vi "add new data to graph.vi"(4 "New Timestamps":timestamp[](array[timestamp]), 7 "Data Array":dbl[](array[numeric]), 8 "Clear Graph":bool, 9 "Max Number of Datapoints":dbl=10000.0 format="%#_13g", 10 "Graph Data":T1(array[cluster])) -> (3 "Graph Data 2":T1(array[cluster]))   [LabVIEW 2013]
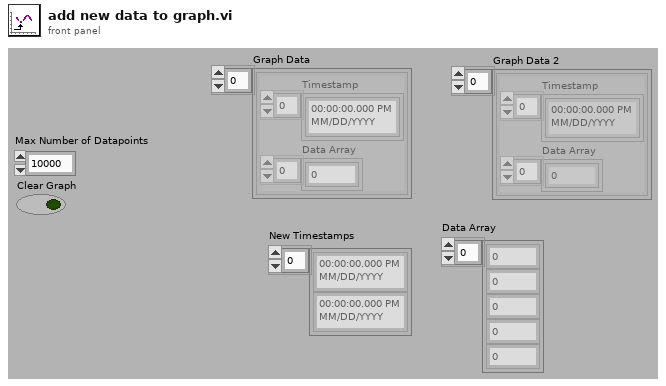
[diagram p1: front panel]
types:
  T1 = cluster{"Timestamp":timestamp[], "Data Array":dbl[]}[]
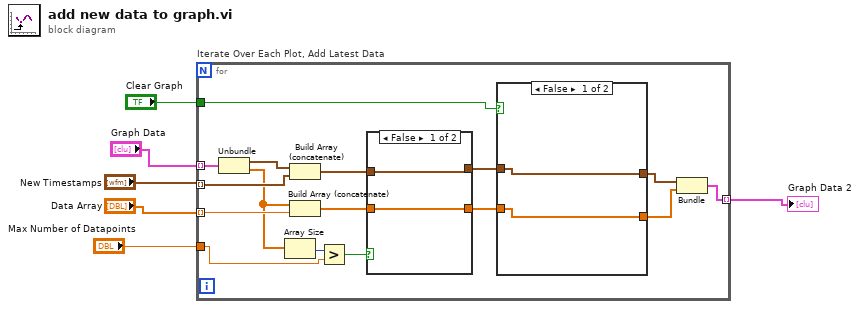
[diagram p0: block diagram]
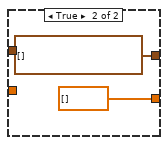
[diagram p2: hidden frame]
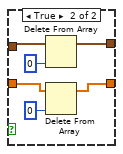
[diagram p3: hidden frame]
diagram:
  n1 = for "Iterate Over Each Plot, Add Latest Data" {
    tunnel: "Graph Data" -> [w22] mode=indexing
    tunnel: "New Timestamps" -> [w18] mode=indexing
    tunnel: "Data Array" -> [w20] mode=indexing
    tunnel: "Max Number of Datapoints" -> [w16]
    tunnel: "Clear Graph" -> [w14]
    tunnel: [w8] -> w5 mode=indexing
    n2 = Unbundle ("Split x and y")(w22) -> ("Timestamp"=w21:timestamp[], "Data Array"=w11:dbl[])
    n3 = Array Size(array=w11) -> (size(s)=w17:i32)
    n4 = Build Array (concatenate) ("Append Latest Values")(w21, w18) -> (w7:timestamp[])
    n5 = Build Array (concatenate)(w11, w20) -> (w19:dbl[])
    n6 = Greater?(x=w17, y=w16) -> (0:w15:bool)
    n7 = case shown="False" w15 {
      tunnel: w19 -> [w27 w32]
      tunnel: w7 -> [w28 w34]
      tunnel: [w28 w30] -> w13
      tunnel: [w27 w29] -> w12
      frame False {
      }
      frame True {
        n8 = Delete From Array(array=w34, index=0) -> (array with subset deleted=w30:timestamp[])  [unwired: 1 in, 1 out]
        n9 = Delete From Array(array=w32, index=0) -> (array with subset deleted=w29:dbl[])  [unwired: 1 in, 1 out]
      }
    }
    n10 = case shown="False" w14 {
      tunnel: [w24 timestamp[] []] -> w10
      tunnel: w13 -> [w24 _]
      tunnel: w12 -> [w23 _]
      tunnel: [w23 dbl[] []] -> w9
      frame False {
      }
      frame True {
      }
    }
    n11 = Bundle(w10, w9) -> (w8:cluster{timestamp[], dbl[]})  [unwired: 1 in]
  }
  "Graph Data 2" <- w5
